vi "AH 2700 Self Test.vi"() -> ()   [LabVIEW 2019]
doc: "This example shows how to configure the bridge to run a self-test and create a report file containing the results."
uses:
  Andeen-Hagerling 2700(400 firmware).lvlib
panel:
  in  "Log Results\nto File":bool
  out "Self-Test Results":string
  in  "VISA Resource":refnum<visa-resource-name>
  in  "Serial Configuration":T1={"Baud Rate"=9600, "Parity"=0, "Data Bits"=8, "Stop Bits"=10} {"Stop Bits" items=["1.0"=10, "1.5"=15, "2.0"=20]; "Data Bits" items=["7"=7, "8"=8]; "Parity" items=["None", "Odd", "Even", "Mark", "Space"]; "Baud Rate" items=["300"=300, "600"=600, "1200"=1200, "2400"=2400, "4800"=4800, "9600"=9600, "19200"=19200, "38400"=38400, "57600"=57600, "115200"=115200]}
  # "AH 2700A ULTRA-PRECISION 50Hz-20kHz CAPACITANCE BRIDGE"
  # "Self Test"
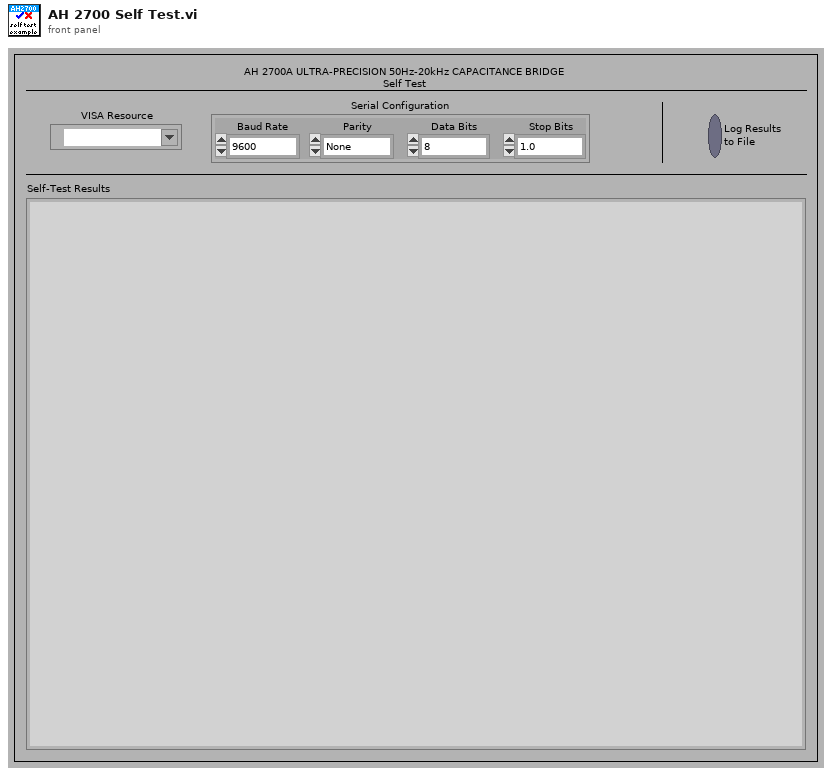
[diagram p1: front panel]
types:
  T1 = cluster{"Baud Rate":u32, "Parity":u16, "Data Bits":u16, "Stop Bits":u16}
  T2 = enum16{"open", "replace", "create", "open or create", "replace or create", "replace or create with confirmation"}
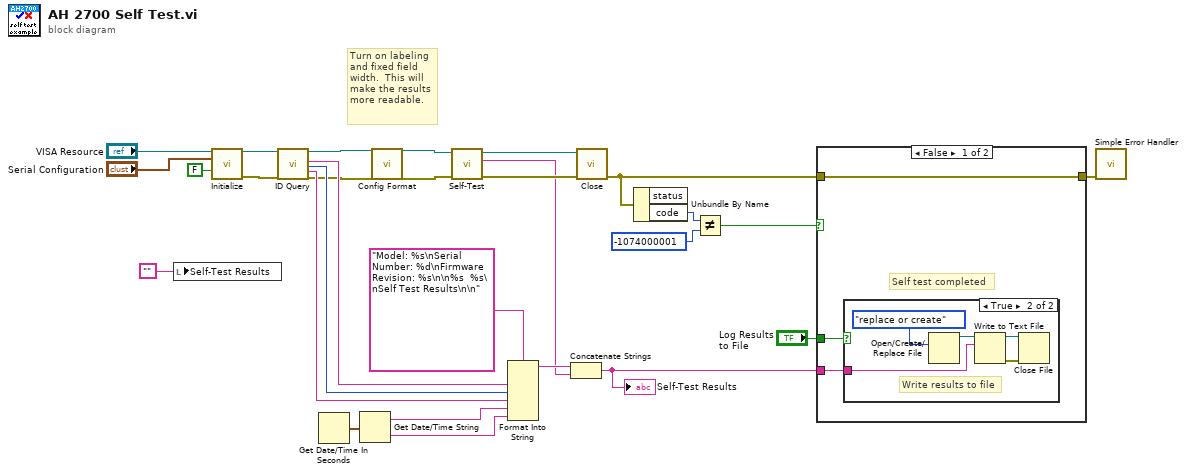
[diagram p0: block diagram]
diagram:
  # "Turn on labeling\nand fixed field\nwidth.  This will\nmake the results\nmore readable."
  n1 = local write "Self-Test Results"("") -> ()
  n2 = call "Initialize.vi"("VISA resource name"="VISA Resource", "Serial Configuration"="Serial Configuration", "Reset (True)"=FALSE) -> ("VISA resource name out"=w6:refnum<visa-resource-name>, "error out"=w5:errorcluster)  [unwired: 11 in]
  n3 = call "ID Query.vi"("VISA resource name"=w6, "error in"=w5) -> ("VISA resource name out"=w10:refnum<visa-resource-name>, "Model Name"=w15:string, "Serial Number"=w14:i32, "Firmware Revision"=w13:string, "error out"=w9:errorcluster)  [unwired: 12 in, 1 out]
  n4 = Get Date/Time In Seconds() -> (seconds since 1Jan1904=w18:timestamp)
  n5 = Get Date/Time String(seconds (now)=w18) -> (date string=w17:string, time string=w16:string)  [unwired: 2 in]
  n6 = call "Config Format.vi"("VISA resource name"=w10, "error in"=w9) -> ("VISA resource name out"=w12:refnum<visa-resource-name>, "error out"=w11:errorcluster)  [unwired: 24 in]
  n7 = call "Self-Test.vi"("error in (no error)"=w11, "VISA resource name"=w12) -> ("error out"=w27:errorcluster, "Self-Test Result Message"=w8:string, "VISA resource name out"=w28:refnum<visa-resource-name>)  [unwired: 6 in, 1 out]
  n8 = Format Into String(format string="Model: %s\nSerial Number: %d\nFirmware Revision: %s\n\n%s  %s\nSelf Test Results\n\n", w15, w14, w13, w17, w16) -> (resulting string=w19:string)  [unwired: 2 in, 1 out]
  n9 = Concatenate Strings(w19, w8) -> (w7:string)
  "Self-Test Results" <- w7
  n10 = call "Close.vi"("error in (no error)"=w27, "VISA resource name"=w28) -> ("error out"=w21:errorcluster)  [unwired: 9 in]
  n11 = Unbundle By Name(w21) -> ("code"=w26:i32)  [unwired: 1 out]
  n12 = Not Equal?(x=w26, y=-1074000001 ("Code")) -> (x != y?=w24:bool)
  n13 = case shown="False" w24 {
    tunnel: "Log Results\nto File" -> [w29 _]
    tunnel: [w31 w37] -> w22
    tunnel: w21 -> [w31 w37]
    tunnel: w7 -> [w30 _]
    frame False {
      # "Self test completed"
      n14 = case shown="True" w29 {
        tunnel: w30 -> [_ w34]
        frame False {
        }
        frame True {
          # "Write results to file"
          n15 = Open/Create/Replace File(operation (0:open)=T2."replace or create") -> (refnum out=w35:refnum<file>)  [unwired: 5 in, 2 out]
          n16 = Write to Text File(file (use dialog)=w35, text=w34) -> (refnum out=w32:refnum<file>, error out=w33:errorcluster)  [unwired: 2 in, 1 out]
          n17 = Close File(refnum=w32, error in=w33) -> ()  [unwired: 2 out]
        }
      }
    }
    frame True {
      # "Self test did not complete.  It encountered an\nerror other than \"self-test failed\"."
    }
  }
  n18 = call <vilib>:"Simple Error Handler.vi"("error in (no error)"=w22) -> ()  [unwired: 4 in, 5 out]
